vi "WindSensorCheckForTimeout.vi"(11 "WindSensorSampleSensorLoopData in":T1) -> (3 "WindSensorSampleSensorLoopData out":T1)   [LabVIEW 2018]
uses:
  WindSensorSampleSensorLoopData.ctl
  WindSensorSampleSensorLoopStates.ctl
  WindSensorSample.ctl
  WindSensorErrorSample.ctl
  WindSensorErrorCodes.ctl
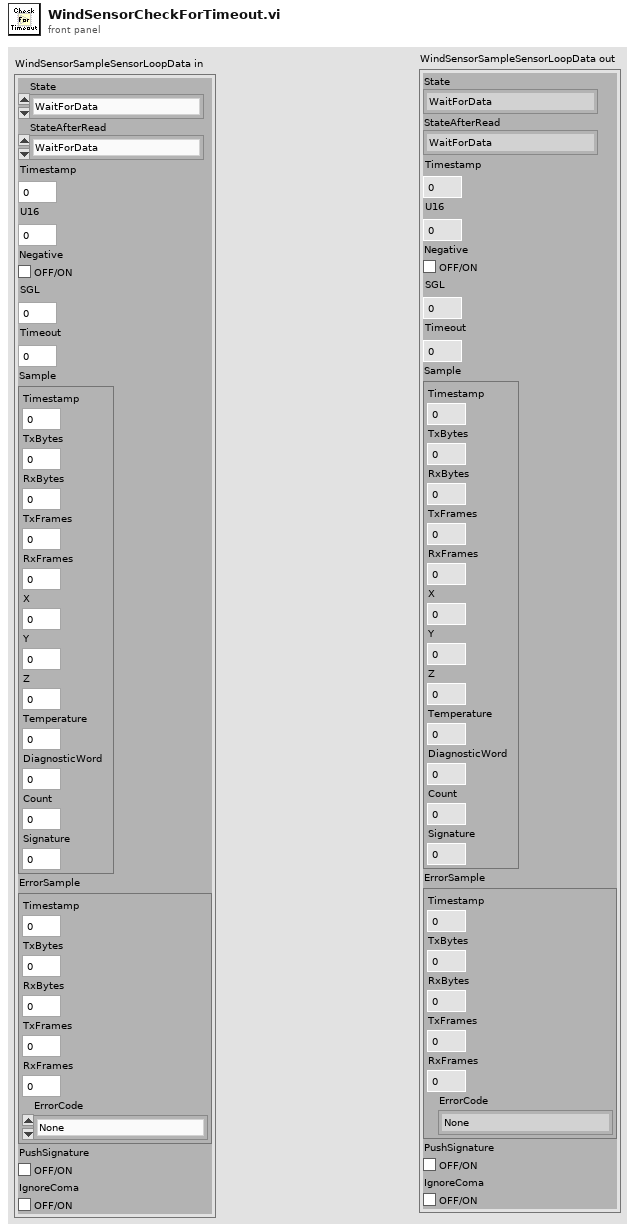
[diagram p1: front panel]
types:
  T1 = typedef "WindSensorSampleSensorLoopData.ctl" = cluster{"State":T2, "StateAfterRead":T2, "Timestamp":u64, "U16":u16, "Negative":bool, "SGL":i32, "Timeout":i32, "Sample":T3, "ErrorSample":T4, "PushSignature":bool, "IgnoreComa":bool}
  T2 = typedef "WindSensorSampleSensorLoopStates.ctl" = enum16{"WaitForData", "StartX", "EndX", "StartY", "EndY", "StartZ", "EndZ", "StartT", "EndT", "StartD", "EndD", "StartC", "EndC", "StartS", "EndS", "CheckSignature", "ReadSGL", "ReadU16", "ReadHexU16", "PrepareSample", "MoveSample", "ResponseUnknownError", "ResponseInvalidError", "ResponseTimeoutError", "ResponseSignatureError", "PrepareErrorCode", "MoveErrorCode", "ClearRxFIFO", "WaitForClearComplete"}
  T3 = typedef "WindSensorSample.ctl" = cluster{"Timestamp":u64, "TxBytes":u64, "RxBytes":u64, "TxFrames":u64, "RxFrames":u64, "X":i32, "Y":i32, "Z":i32, "Temperature":i32, "DiagnosticWord":u16, "Count":u8, "Signature":u16}
  T4 = typedef "WindSensorErrorSample.ctl" = cluster{"Timestamp":u64, "TxBytes":u64, "RxBytes":u64, "TxFrames":u64, "RxFrames":u64, "ErrorCode":T5}
  T5 = typedef "WindSensorErrorCodes.ctl" = enum16{"None", "ResponseUnknownError", "ResponseInvalidError", "ResponseTimeoutError", "ResponseSignatureError"}
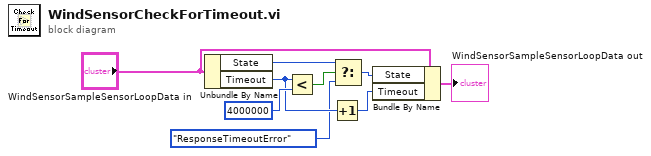
[diagram p0: block diagram]
diagram:
  n1 = Unbundle By Name("WindSensorSampleSensorLoopData in") -> ("State"=w1:T2, "Timeout"=w7:i32)
  n2 = Less?(x=w7, y=4000000) -> (x < y?=w8:bool)
  n3 = Increment(x=w7) -> (x+1=w2:i32)
  n4 = Select(t=w1, s=w8, f=WindSensorSampleSensorLoopStates."ResponseTimeoutError") -> (s? t:f=w3:T2)
  n5 = Bundle By Name(cluster="WindSensorSampleSensorLoopData in", "State"=w3, "Timeout"=w2) -> (→"WindSensorSampleSensorLoopData out":T1)
